vi "更新IOT扭力数据.vi"(8 "前/后":bool) -> ()   [LabVIEW 2017]
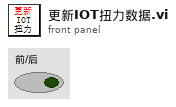
[diagram p1: front panel]
types:
  T1 = typedef "IOT数据更新选项.ctl" = enum16{"初始化", "更新数据", "获取寄存器", "前后站信息交互", "更新前站inflow&barcode"}
  T2 = typedef "螺丝机IOT数据信息.ctl" = cluster{"IOT基本信息":T3, "扭力":string[]}
  T3 = typedef "IOT数据基本信息.ctl" = cluster{"number":string, "ID":string, "Version":string, "Date":string, "Time":string, "Device SN":string, "Carrier SN":string, "Inflow":string, "Work":string, "Wait":string, "Outflow":string, "SFIS":string, "Alignment Times":string, "Press1":string, "ifsyn":string}
  T4 = typedef "模块操作选项.ctl" = enum16{"初始化", "更新起子&扭力", "旋转操作", "获取寄存器"}
  T5 = typedef "提取参数项目.ctl" = enum16{"初始化", "基准拍照点提取", "物理距离信息提取", "锁附总表参数提取", "图纸锁附坐标提取", "更新图面offset", "图纸投影至机械", "提取数据"}
  T6 = typedef "起子部分集合输出.ctl" = cluster{"扭力&速度反馈量":T7[], "计算后输出量":T8[], "当前起子参数":T9[]}
  T7 = typedef "转矩&速度.ctl" = cluster{"转矩量":dbl, "转速量":dbl}
  T8 = typedef "起子计算输出集合.ctl" = cluster{"转矩&速度输出":T7, "扭力达到信号":bool}
  T9 = typedef "设置参数.ctl" = cluster{"惯量比":sgl, "输入扭力":sgl, "转速最大限制":sgl}
  T10 = typedef "起子编号.ctl" = enum16{"NA", "driver01", "driver02", "driver03", "driver04"}
  T11 = typedef "参数集合.ctl" = cluster{"主&辅助定位孔拍照位置":T12, "物距提取信息":T14, "锁附总表参数":T17, "图面投影后检索结果":T21}
  T12 = typedef "主&辅助定位孔拍照位置.ctl" = cluster{"主定位孔拍照位置":T13, "辅助定位孔拍照位置":T13}
  T13 = typedef "定位孔拍照位置.ctl" = cluster{"动子位置":dbl, "供料轴位置":dbl, "Z轴位置":dbl}
  T14 = typedef "物距提取信息.ctl" = cluster{"物距":T15, "橡皮泥标记点":T13, "物距文档检索状态":T16, "标记拍照Z轴":dbl}
  T15 = typedef "物理距离.ctl" = cluster{"动子方向":dbl, "供料轴方向":dbl}
  T16 = typedef "总表检索状态.ctl" = enum16{"检索点位顺序超出范围", "检索OK"}
  T17 = typedef "锁附参数.ctl" = cluster{"锁附扭力":dbl, "锁附位置参数":T18, "锁附速度":T19, "锁附检测类参数":T20, "锁附点位编号":string, "总表检索状态":T16, "锁附总颗数":dbl, "起子编号":T10, "顺序编号":dbl, "组装孔？":bool, "扭力offset":dbl, "设定扭力":dbl, "锁附自救屏蔽？":bool}
  T18 = typedef "锁附位置参数.ctl" = cluster{"动子位置":dbl, "供料轴位置":dbl, "阶梯高度位置":dbl, "锁附深度":dbl}
  T19 = typedef "锁附速度.ctl" = cluster{"驱动速度":dbl, "加速度":dbl}
  T20 = typedef "锁附检测类参数.ctl" = cluster{"报警功能屏蔽？":bool, "锁附设定时间":dbl, "浮锁检测高度":dbl, "浮锁检测容差":dbl}
  T21 = typedef "图面投影后检索结果.ctl" = cluster{"图纸投影后点位坐标":T15, "图面投影后文件检索状态":T16, "offset获取辅助集合":T22}
  T22 = typedef "offset获取辅助集合.ctl" = cluster{"offset获取半径spec":T23, "拍照高度":dbl, "曝光时间":dbl}
  T23 = typedef "上下限.ctl" = cluster{"上限":dbl, "下限":dbl}
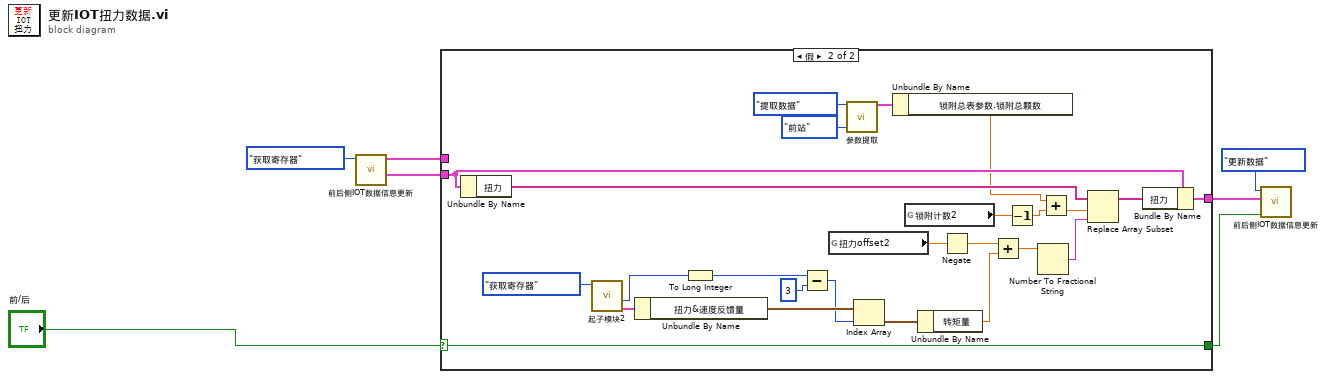
[diagram p0: block diagram]
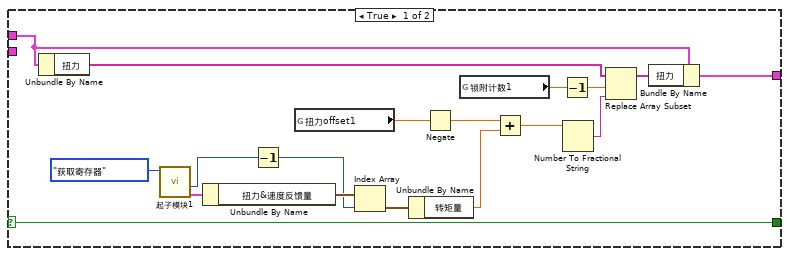
[diagram p2: hidden frame]
diagram:
  n1 = call "前后侧IOT数据信息更新.vi"("选项"=IOT数据更新选项."获取寄存器") -> ("后侧IOT数据信息"=w6:T2, "前侧IOT数据信息"=w3:T2)  [unwired: 9 in]
  n2 = case shown="假" "前/后" {
    selector: "前/后" -> [w8 w37]
    tunnel: w3 -> [w16 _]
    tunnel: [w9 w38] -> w4
    tunnel: [w8 w37] -> w5
    tunnel: w6 -> [_ w31]
    frame True {
      n3 = Unbundle By Name(w16) -> ("扭力"=w15:string[])
      n4 = call "起子模块1.vi"("模块操作选项"=模块操作选项."获取寄存器") -> ("起子部分集合输出"=w24:T6, "锁附起子编号out"=w22:T10)  [unwired: 8 in, 1 out]
      n5 = Unbundle By Name(w24) -> ("扭力&速度反馈量"=w23:T7[])
      n6 = Decrement(x=w22) -> (x-1=w21:T10)
      n7 = global read "流程全局.vi" "扭力offset1"() -> (w19:dbl)
      n8 = Index Array(array=w23, index=w21) -> (element=w20:T7)
      n9 = Unbundle By Name(w20) -> ("转矩量"=w18:dbl)
      n10 = Negate(x=w19) -> (-x=w17:dbl)
      n11 = global read "流程全局.vi" "锁附计数1"() -> (w11:dbl)
      n12 = Add(x=w17, y=w18) -> (x+y=w14:dbl)
      n13 = Decrement(x=w11) -> (x-1=w10:dbl)
      n14 = Number To Fractional String(number=w14) -> (F-format string=w13:string)  [unwired: 3 in]
      n15 = Replace Array Subset(array=w15, new element=w13, index=w10) -> (w12:string[])
      n16 = Bundle By Name(cluster=w16, "扭力"=w12) -> (w9:T2)
    }
    frame False {
      n17 = Unbundle By Name(w31) -> ("扭力"=w44:string[])
      n18 = call "起子模块2.vi"("模块操作选项"=模块操作选项."获取寄存器") -> ("起子部分集合输出"=w34:T6, "锁附起子编号out"=w35:T10)  [unwired: 8 in, 1 out]
      n19 = Unbundle By Name(w34) -> ("扭力&速度反馈量"=w50:T7[])
      n20 = To Long Integer(number=w35) -> (32bit integer=w33:i32)
      n21 = Subtract(x=w33, y=3 ("x")) -> (x-y=w49:i32)
      n22 = global read "流程全局.vi" "扭力offset2"() -> (w47:dbl)
      n23 = call "参数提取.vi"("提取参数项目"=提取参数项目."提取数据", "前/后站"=enum16{"前站", "后站"}."前站") -> ("参数集合out"=w28:T11)  [unwired: 10 in, 3 out]
      n24 = Index Array(array=w50, index=w49) -> (element=w48:T7)
      n25 = Unbundle By Name(w28) -> ("锁附总表参数.锁附总颗数"=w26:dbl)
      n26 = global read "流程全局.vi" "锁附计数2"() -> (w40:dbl)
      n27 = Unbundle By Name(w48) -> ("转矩量"=w46:dbl)
      n28 = Negate(x=w47) -> (-x=w45:dbl)
      n29 = Add(x=w45, y=w46) -> (x+y=w43:dbl)
      n30 = Decrement(x=w40) -> (x-1=w39:dbl)
      n31 = Number To Fractional String(number=w43) -> (F-format string=w42:string)  [unwired: 3 in]
      n32 = Add(x=w26, y=w39) -> (x+y=w27:dbl)
      n33 = Replace Array Subset(array=w44, new element=w42, index=w27) -> (w41:string[])
      n34 = Bundle By Name(cluster=w31, "扭力"=w41) -> (w38:T2)
    }
  }
  n35 = call "前后侧IOT数据信息更新.vi"("前/后侧"=w5, "IOT数据信息"=w4, "选项"=IOT数据更新选项."更新数据") -> ()  [unwired: 7 in, 2 out]
